vi "SetPanelPosion.vi"(8 "Bottom":i16, 9 "Right":i16, 11 "VI ref in":refnum<vi>) -> (3 "VI ref out":refnum<vi>)   [LabVIEW 2015]
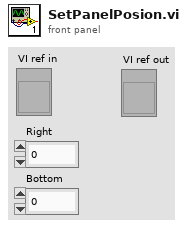
[diagram p1: front panel]
types:
  T1 = typedef "LVRectTypeDef.ctl" = cluster{"Left":i16, "Top":i16, "Right":i16, "Bottom":i16}
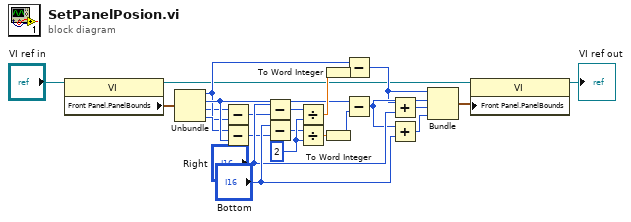
[diagram p0: block diagram]
diagram:
  w20 = i16 2 ("y")
  n1 = property class="VI"(reference="VI ref in") -> (reference out=w4:refnum<vi>, "Front Panel.PanelBounds"=w3:T1)  [unwired: 1 in, 1 out]
  n2 = Unbundle(w3) -> ("Left"=w11:i16, "Top"=w13:i16, "Right"=w10:i16, "Bottom"=w12:i16)
  n3 = Subtract(x=w10, y=w11) -> (x-y=w14:i16)
  n4 = Subtract(x=w12, y=w13) -> (x-y=w15:i16)
  n5 = Subtract(x="Right", y=w14) -> (x-y=w18:i16)
  n6 = Subtract(x="Bottom", y=w15) -> (x-y=w19:i16)
  n7 = Divide(x=w18, y=w20) -> (x/y=w21:dbl)
  n8 = Divide(x=w19, y=w20) -> (x/y=w22:dbl)
  n9 = To Word Integer(number=w21) -> (16bit integer=w24:i16)
  n10 = To Word Integer(number=w22) -> (16bit integer=w23:i16)
  n11 = Subtract(x=w11, y=w24) -> (x-y=w8:i16)
  n12 = Subtract(x=w13, y=w23) -> (x-y=w9:i16)
  n13 = Add(x=w8, y="Right") -> (x+y=w6:i16)
  n14 = Add(x=w9, y="Bottom") -> (x+y=w5:i16)
  n15 = Bundle(w8, w9, w6, w5) -> (w7:cluster{i16, i16, i16, i16})  [unwired: 1 in]
  n16 = property class="VI"(reference=w4, "Front Panel.PanelBounds"=w7) -> (reference out=→"VI ref out":refnum<vi>)  [unwired: 1 in, 1 out]
